vi "IMU Complementary Filter.vi"(7 "dt (ms)":u16, 9 "Accelerometer Angle":dbl, 11 "Angular vel (gyro, deg/sec)":dbl) -> (2 "Current Angle":dbl)   [LabVIEW 2014]
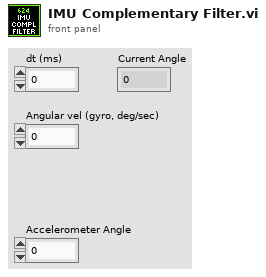
[diagram p1: front panel]
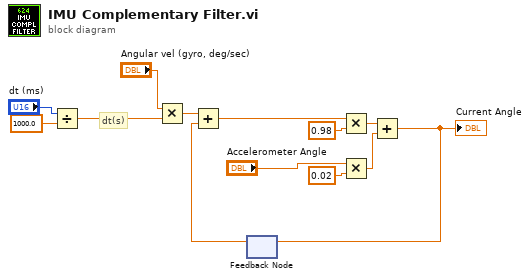
[diagram p0: block diagram]
diagram:
  # "dt(s)"
  n1 = Divide(x="dt (ms)", y=1000.0) -> (x/y=w1:dbl)
  n2 = Multiply(x="Angular vel (gyro, deg/sec)", y=w1) -> (x*y=w13:dbl)
  n3 = feedback #1() -> (w5:dbl)  [unwired: 1 in]
  n4 = Add(x=w13, y=w5) -> (x+y=w6:dbl)
  n5 = Multiply(x=w6, y=0.98) -> (x*y=w11:dbl)
  n6 = Multiply(x="Accelerometer Angle", y=0.02) -> (x*y=w12:dbl)
  n7 = Add(x=w11, y=w12) -> (x+y=w4:dbl)
  "Current Angle" <- w4
  n8 = feedback-in #1(w4) -> ()
